vi "remove.issue.vi"(8 "error in":errorcluster, 9 "issue ids":i32[](array[numeric]), 11 "manager_daemon in":refnum<class "manager_daemon.lvclass">) -> (0 "error out":errorcluster, 3 "manager_daemon out":refnum<class "manager_daemon.lvclass">)   [LabVIEW 2024, in "manager_daemon.lvclass"]
uses:
  manager_daemon.lvclass
  manager_daemon.lvclass/manager_daemon.ctl
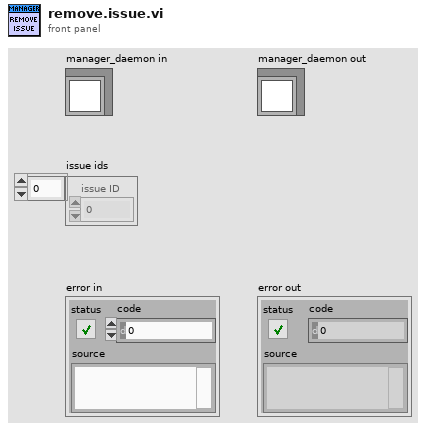
[diagram p1: front panel]
types:
  T1 = typedef "manager_daemon.lvclass/VolumeData--cluster.ctl" = cluster{"name":string, "sortable_name":string, "aliases":string[], "description":string, "site_detail_url":string, "count_of_issues":i32, "start_year":i32, "publisher_id":i32, "issue_ids":i32[], "date_last_updated":timestamp, "volume":i32, "cv_id":string, "volume type":T2, "source_path":path}
  T2 = typedef "CV_Shared_Library.lvlib/volume.type--enum.ctl" = enum16{"Ongoing", "Limited Series", "Annual", "One Shot", "Reprint/Document", "Star Comics", "Epic Comics"}
  T3 = typedef "manager_daemon.lvclass/sub-map--map.ctl" = map{string, T4}
  T4 = typedef "manager_daemon.lvclass/SubData--cluster.ctl" = cluster{"id":i32, "issues":set{i32}}
  T5 = typedef "manager_daemon.lvclass/IssueData--clustrer.ctl" = cluster{"cover_date":timestamp, "cv_id":string, "name":string, "sortable_name":string, "issue_number":string, "deck":string, "description":string, "id":i32, "store_date":timestamp, "date_last_updated":timestamp, "site_detail_url":string, "cover_url":string, "source_path":path}
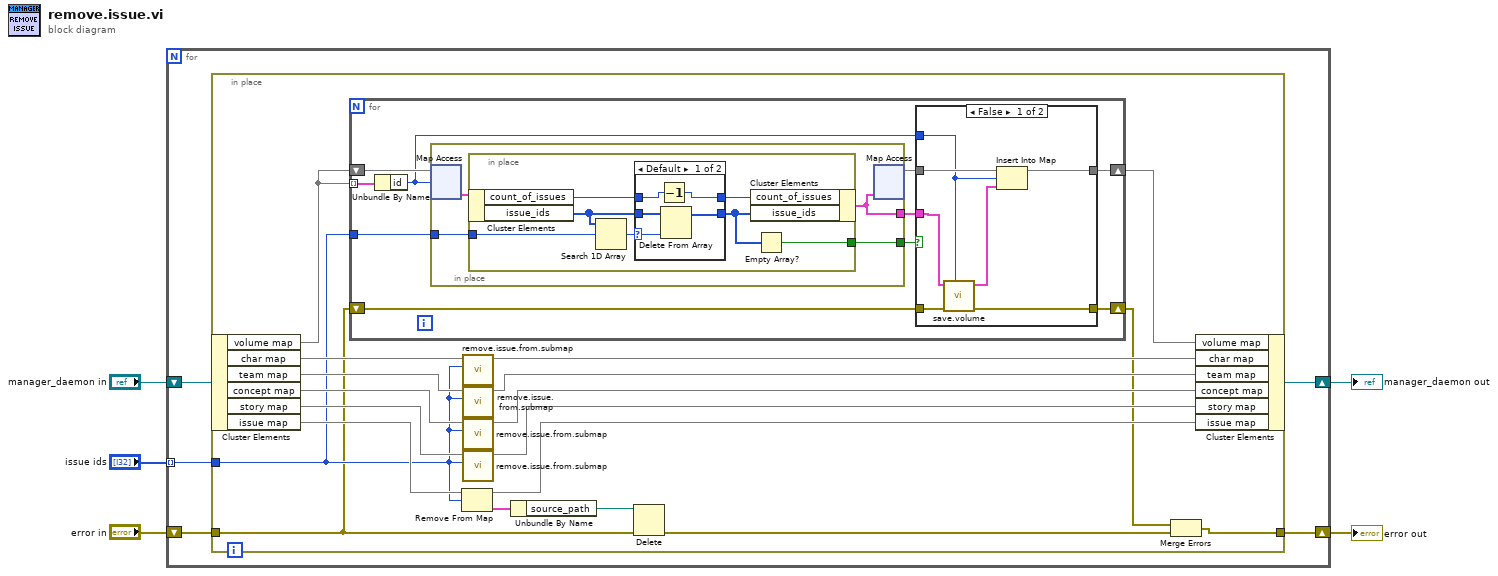
[diagram p0: block diagram]
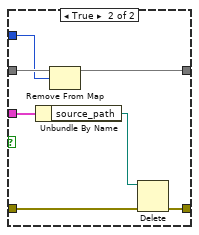
[diagram p3: hidden frame]
diagram:
  n1 = for {
    tunnel: "issue ids" -> [w8] mode=indexing
    shift-right: [w9] -> w3
    shift-left: "manager_daemon in" -> [w10]
    shift-right: [w6] -> w1
    shift-left: "error in" -> [w7]
    n2 = in-place {
      in-place-border: w8 -> [w18]
      in-place-border: w7 -> [w14]
      in-place-border: [w11] -> w6
      n3 = in-place-cluster #1(w10) -> ("volume map"=w21:map{i32, T1}, "char map"=w29:T3, "team map"=w27:T3, "concept map"=w26:T3, "story map"=w25:T3, "issue map"=w19:map{i32, T5})
      n4 = for {
        tunnel: w21 -> [w39] mode=indexing
        tunnel: w18 -> [w37]
        shift-right: [w34] -> w20
        shift-left: w21 -> [w38]
        shift-right: [w31] -> w12
        shift-left: w14 -> [w32]
        n5 = Unbundle By Name(w39) -> ("id"=w33:i32)
        n6 = in-place {
          in-place-border: w37 -> [w42]
          in-place-border: [w41] -> w36
          in-place-border: [w40] -> w30
          n7 = in-place-map #2(w38, w33) -> (w43:T1)  [unwired: 1 in, 1 out]
          n8 = in-place {
            in-place-border: w42 -> [w50]
            in-place-border: [w46] -> w41
            n9 = in-place-cluster #3(w43) -> ("count_of_issues"=w45:i32, "issue_ids"=w48:i32[])
            n10 = Search 1D Array(1D array=w48, element=w50) -> (index of element=w49:i32)  [unwired: 1 in]
            n11 = case shown="Default" w49 {
              selector: w49 -> [w55 _]
              tunnel: [w53 w57] -> w47
              tunnel: w48 -> [w54 w57]
              tunnel: w45 -> [w52 w56]
              tunnel: [w51 w56] -> w44
              frame Default {
                n12 = Decrement(x=w52) -> (x-1=w51:i32)
                n13 = Delete From Array(array=w54, index=w55) -> (array with subset deleted=w53:i32[])  [unwired: 1 in, 1 out]
              }
              frame -1 {
              }
            }
            n14 = in-place-cluster #3("count_of_issues"=w44, "issue_ids"=w47) -> (w40:T1)
            n15 = Empty Array?(array=w47) -> (empty?=w46:bool)
          }
          n16 = in-place-map #2(w40) -> (w35:map{i32, T1})  [unwired: 1 in, 2 out]
        }
        n17 = case shown="False" w36 {
          tunnel: w35 -> [w61 w71]
          tunnel: [w58 w70] -> w34
          tunnel: w33 -> [w59 w69]
          tunnel: w32 -> [w64 w68]
          tunnel: [w62 w67] -> w31
          tunnel: w30 -> [w63 w66]
          frame False {
            n18 = call "save.volume.vi"("id"=w59, "error in (no error)"=w64, "volume"=w63) -> ("error out"=w62:errorcluster, "volume out"=w60:T1)  [unwired: 7 in]
            n19 = Insert Into Map(map in=w61, key=w59, value=w60) -> (map out=w58:map{i32, T1})  [unwired: 2 out]
          }
          frame True {
            n20 = Unbundle By Name(w66) -> ("source_path"=w65:path)
            n21 = Remove From Map(10:w69, 11:w71) -> (3:w70:map{i32, T1})  [unwired: 2 out]
            n22 = Delete(path (use dialog)=w65, error in=w68) -> (error out=w67:errorcluster)  [unwired: 3 in, 2 out]
          }
        }
      }
      n23 = Remove From Map(10:w18, 11:w19) -> (1:w16:T5, 3:w17:map{i32, T5})  [unwired: 1 out]
      n24 = call "remove.issue.from.submap.vi"("issue id"=w18, "map in"=w29) -> ("map out"=w28:T3)  [unwired: 9 in]
      n25 = call "remove.issue.from.submap.vi"("issue id"=w18, "map in"=w27) -> ("map out"=w24:T3)  [unwired: 9 in]
      n26 = call "remove.issue.from.submap.vi"("issue id"=w18, "map in"=w26) -> ("map out"=w23:T3)  [unwired: 9 in]
      n27 = call "remove.issue.from.submap.vi"("issue id"=w18, "map in"=w25) -> ("map out"=w22:T3)  [unwired: 9 in]
      n28 = Unbundle By Name(w16) -> ("source_path"=w15:path)
      n29 = Delete(path (use dialog)=w15, error in=w14) -> (error out=w13:errorcluster)  [unwired: 3 in, 2 out]
      n30 = Merge Errors(w12, w13) -> (w11:errorcluster)
      n31 = in-place-cluster #1("volume map"=w20, "char map"=w28, "team map"=w24, "concept map"=w23, "story map"=w22, "issue map"=w17) -> (w9:refnum<class "manager_daemon.lvclass">)
    }
  }
  "manager_daemon out" <- w3
  "error out" <- w1
